vi "Reply.vi"(8 "error in (no error)":errorcluster, 10 "Response":string, 11 "MicronMessage in":refnum<class "Message.lvclass">) -> (0 "error out":errorcluster, 3 "MicronMessage out":refnum<class "Message.lvclass">)   [LabVIEW 2019, in "Micron.lvlib" / "Message.lvclass"]
uses:
  Message.lvclass
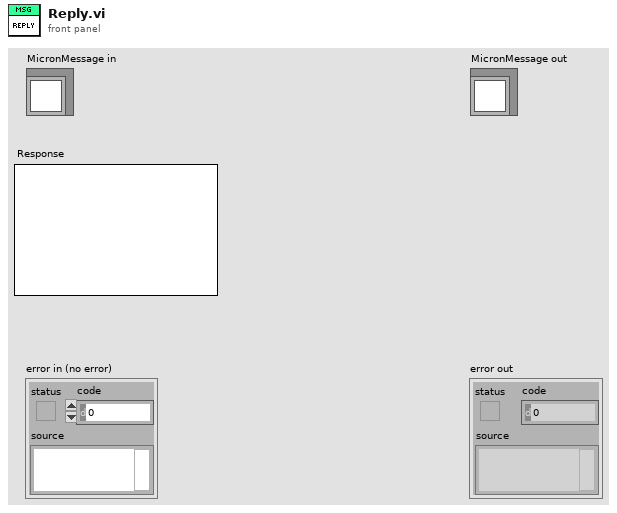
[diagram p1: front panel]
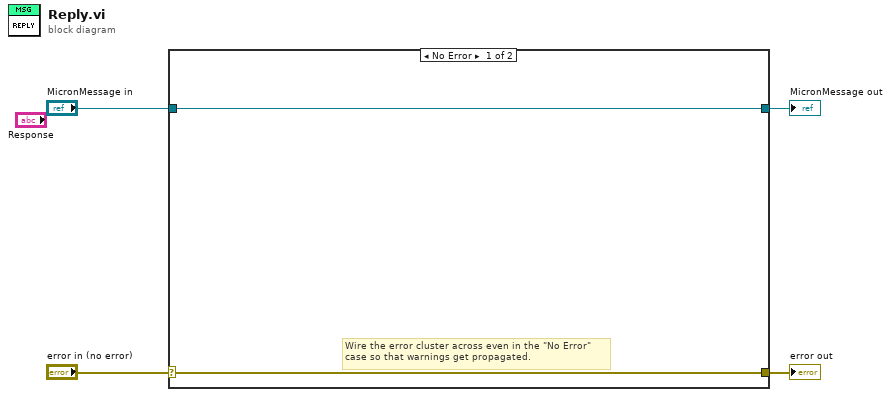
[diagram p0: block diagram]
diagram:
  n1 = case shown="No Error" "error in (no error)" {
    selector: "error in (no error)" -> [w5 w8]
    tunnel: [w5 w8] -> w3
    tunnel: [w6 w7] -> w1
    tunnel: "MicronMessage in" -> [w6 w7]
    frame No Error {
      # "Wire the error cluster across even in the \"No Error\"\ncase so that warnings get propagated."
    }
    frame Error {
    }
  }
  "error out" <- w3
  "MicronMessage out" <- w1
